vi "Read Dashboard Variables.vi"() -> ()   [LabVIEW 2018]
uses:
  <vilib>/Rock Robotics/Network Tables/NT Read Number.vi
  Framework/Robot Global Data.vi
panel:
  out "Elevator Cargo":dbl=2.0
  out "Elevator Hatch 3":dbl=2.0
  out "Elevator Hatch 2":dbl=2.0
  out "Elevator Hatch 1":dbl=2.0
  out "Elevator Ball 3":dbl=2.0
  out "Elevator Ball 2":dbl=2.0
  out "Elevator Ball 1":dbl=2.0
  out "Hatch Mover Scale":dbl=1.0 min=0.0 max=1.0 step=0.1
  out "Elevator Scale":dbl=1.0 min=0.0 max=1.0 step=0.1
  out "Autonomous Wait":u32=10
  out "Hatch Mover Duration":dbl=3.0
  out "Hatch Mover Setpoint":dbl=1.0
  out "SlowModeSettings":i32=2
  out "MaxSpeedSlow":dbl=0.4
  out "SlowRate":dbl=1.0
  out "MaxTurnSlow":dbl=0.55
  out "MaxTurnRateSlow":dbl=20.0
  out "Cargo Stop Current":dbl=10.0
  out "Cargo Hold Duration":dbl=1.0
  out "Cheezy Drive Mode":u32=2
  out "Cargo Setpoint":dbl=1.0 min=0.0 max=1.0 step=0.1
  out "Elevator Duration":dbl=2.0
  out "Elevator Setpoint":dbl=1.0 min=0.0 max=1.0 step=0.1
  out "Pivot Right Setpoint":dbl=0.3 min=0.0 max=1.0 step=0.1
  out "Pivot Left Setpoint":dbl=0.3 min=0.0 max=1.0 step=0.1
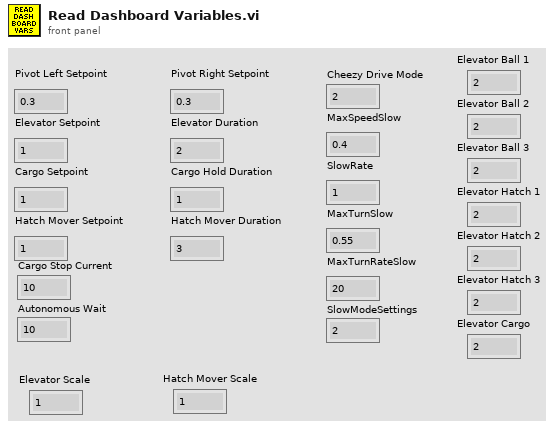
[diagram p1: front panel]
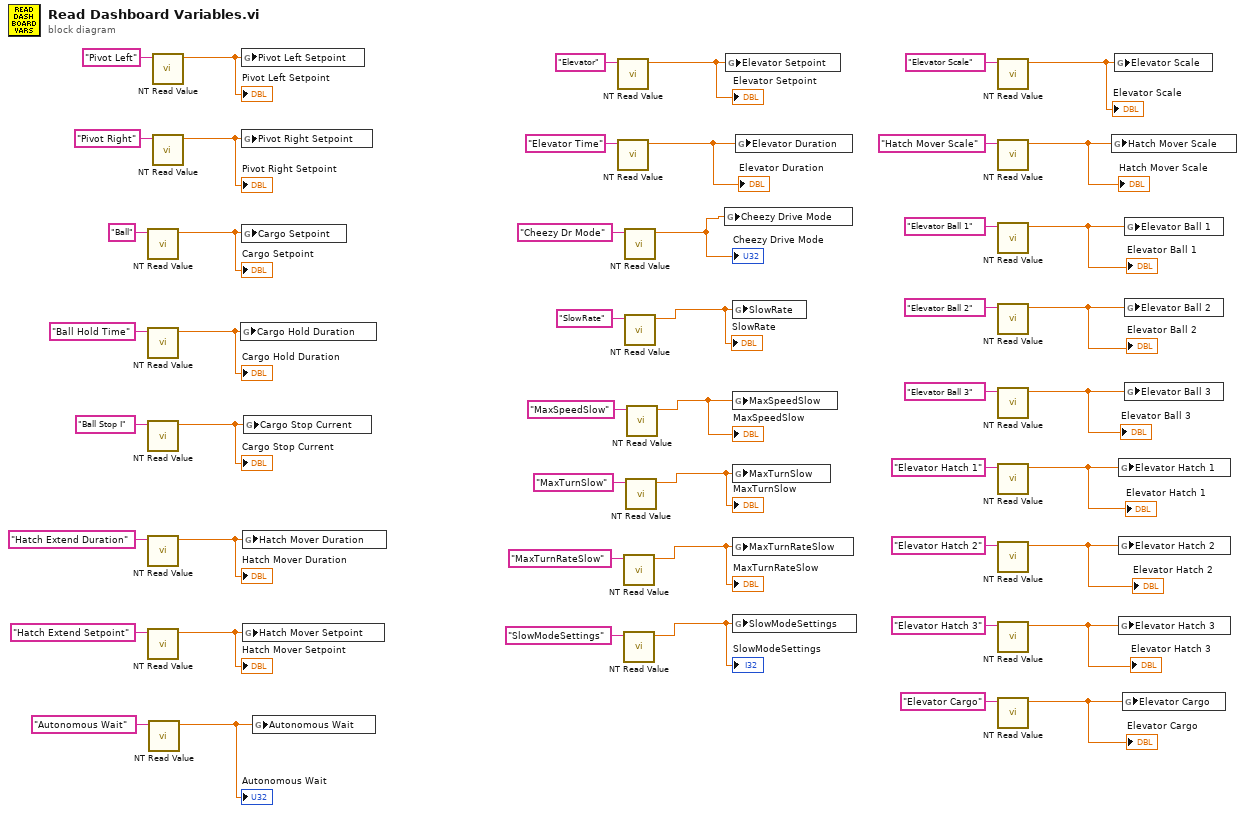
[diagram p0: block diagram]
diagram:
  n1 = call-poly <vilib>:"NT Read Value.vi"("Name"="Ball") -> ("Numeric"=w33:dbl)  [unwired: 9 in, 1 out]
  "Cargo Setpoint" <- w33
  n2 = call-poly <vilib>:"NT Read Value.vi"("Name"="Ball Hold Time") -> ("Numeric"=w32:dbl)  [unwired: 9 in, 1 out]
  "Cargo Hold Duration" <- w32
  n3 = call-poly <vilib>:"NT Read Value.vi"("Name"="Ball Stop I") -> ("Numeric"=w31:dbl)  [unwired: 9 in, 1 out]
  "Cargo Stop Current" <- w31
  n4 = call-poly <vilib>:"NT Read Value.vi"("Name"="Hatch Extend Duration") -> ("Numeric"=w30:dbl)  [unwired: 9 in, 1 out]
  "Hatch Mover Duration" <- w30
  n5 = call-poly <vilib>:"NT Read Value.vi"("Name"="Hatch Extend Setpoint") -> ("Numeric"=w29:dbl)  [unwired: 9 in, 1 out]
  "Hatch Mover Setpoint" <- w29
  n6 = call-poly <vilib>:"NT Read Value.vi"("Name"="Autonomous Wait") -> ("Numeric"=w20:dbl)  [unwired: 9 in, 1 out]
  "Autonomous Wait" <- w20
  n7 = call-poly <vilib>:"NT Read Value.vi"("Name"="Pivot Left") -> ("Numeric"=w35:dbl)  [unwired: 9 in, 1 out]
  "Pivot Left Setpoint" <- w35
  n8 = call-poly <vilib>:"NT Read Value.vi"("Name"="Pivot Right") -> ("Numeric"=w34:dbl)  [unwired: 9 in, 1 out]
  "Pivot Right Setpoint" <- w34
  n9 = global write "Robot Global Data.vi" "Cargo Hold Duration"(w32) -> ()
  n10 = global write "Robot Global Data.vi" "Pivot Left Setpoint"(w35) -> ()
  n11 = global write "Robot Global Data.vi" "Pivot Right Setpoint"(w34) -> ()
  n12 = global write "Robot Global Data.vi" "Cargo Setpoint"(w33) -> ()
  n13 = global write "Robot Global Data.vi" "Hatch Mover Duration"(w30) -> ()
  n14 = global write "Robot Global Data.vi" "Hatch Mover Setpoint"(w29) -> ()
  n15 = global write "Robot Global Data.vi" "Cargo Stop Current"(w31) -> ()
  n16 = global write "Robot Global Data.vi" "Autonomous Wait"(w20) -> ()
  n17 = call-poly <vilib>:"NT Read Value.vi"("Name"="Elevator") -> ("Numeric"=w22:dbl)  [unwired: 9 in, 1 out]
  "Elevator Setpoint" <- w22
  n18 = call-poly <vilib>:"NT Read Value.vi"("Name"="Elevator Time") -> ("Numeric"=w8:dbl)  [unwired: 9 in, 1 out]
  "Elevator Duration" <- w8
  n19 = call-poly <vilib>:"NT Read Value.vi"("Name"="MaxTurnRateSlow") -> ("Numeric"=w24:dbl)  [unwired: 9 in, 1 out]
  "MaxTurnRateSlow" <- w24
  n20 = call-poly <vilib>:"NT Read Value.vi"("Name"="SlowModeSettings") -> ("Numeric"=w23:dbl)  [unwired: 9 in, 1 out]
  "SlowModeSettings" <- w23
  n21 = call-poly <vilib>:"NT Read Value.vi"("Name"="Cheezy Dr Mode") -> ("Numeric"=w28:dbl)  [unwired: 9 in, 1 out]
  "Cheezy Drive Mode" <- w28
  n22 = call-poly <vilib>:"NT Read Value.vi"("Name"="SlowRate") -> ("Numeric"=w27:dbl)  [unwired: 9 in, 1 out]
  "SlowRate" <- w27
  n23 = call-poly <vilib>:"NT Read Value.vi"("Name"="MaxTurnSlow") -> ("Numeric"=w25:dbl)  [unwired: 9 in, 1 out]
  "MaxTurnSlow" <- w25
  n24 = call-poly <vilib>:"NT Read Value.vi"("Name"="MaxSpeedSlow") -> ("Numeric"=w26:dbl)  [unwired: 9 in, 1 out]
  "MaxSpeedSlow" <- w26
  n25 = global write "Robot Global Data.vi" "Cheezy Drive Mode"(w28) -> ()
  n26 = global write "Robot Global Data.vi" "Elevator Setpoint"(w22) -> ()
  n27 = global write "Robot Global Data.vi" "SlowRate"(w27) -> ()
  n28 = global write "Robot Global Data.vi" "MaxSpeedSlow"(w26) -> ()
  n29 = global write "Robot Global Data.vi" "MaxTurnSlow"(w25) -> ()
  n30 = global write "Robot Global Data.vi" "MaxTurnRateSlow"(w24) -> ()
  n31 = global write "Robot Global Data.vi" "SlowModeSettings"(w23) -> ()
  n32 = global write "Robot Global Data.vi" "Elevator Duration"(w8) -> ()
  n33 = call-poly <vilib>:"NT Read Value.vi"("Name"="Elevator Scale") -> ("Numeric"=w17:dbl)  [unwired: 9 in, 1 out]
  "Elevator Scale" <- w17
  n34 = call-poly <vilib>:"NT Read Value.vi"("Name"="Hatch Mover Scale") -> ("Numeric"=w16:dbl)  [unwired: 9 in, 1 out]
  "Hatch Mover Scale" <- w16
  n35 = call-poly <vilib>:"NT Read Value.vi"("Name"="Elevator Ball 1") -> ("Numeric"=w7:dbl)  [unwired: 9 in, 1 out]
  "Elevator Ball 1" <- w7
  n36 = call-poly <vilib>:"NT Read Value.vi"("Name"="Elevator Ball 2") -> ("Numeric"=w6:dbl)  [unwired: 9 in, 1 out]
  "Elevator Ball 2" <- w6
  n37 = call-poly <vilib>:"NT Read Value.vi"("Name"="Elevator Ball 3") -> ("Numeric"=w5:dbl)  [unwired: 9 in, 1 out]
  "Elevator Ball 3" <- w5
  n38 = call-poly <vilib>:"NT Read Value.vi"("Name"="Elevator Hatch 1") -> ("Numeric"=w4:dbl)  [unwired: 9 in, 1 out]
  "Elevator Hatch 1" <- w4
  n39 = call-poly <vilib>:"NT Read Value.vi"("Name"="Elevator Hatch 2") -> ("Numeric"=w3:dbl)  [unwired: 9 in, 1 out]
  "Elevator Hatch 2" <- w3
  n40 = call-poly <vilib>:"NT Read Value.vi"("Name"="Elevator Hatch 3") -> ("Numeric"=w2:dbl)  [unwired: 9 in, 1 out]
  "Elevator Hatch 3" <- w2
  n41 = call-poly <vilib>:"NT Read Value.vi"("Name"="Elevator Cargo") -> ("Numeric"=w1:dbl)  [unwired: 9 in, 1 out]
  "Elevator Cargo" <- w1
  n42 = global write "Robot Global Data.vi" "Hatch Mover Scale"(w16) -> ()
  n43 = global write "Robot Global Data.vi" "Elevator Scale"(w17) -> ()
  n44 = global write "Robot Global Data.vi" "Elevator Hatch 1"(w4) -> ()
  n45 = global write "Robot Global Data.vi" "Elevator Hatch 2"(w3) -> ()
  n46 = global write "Robot Global Data.vi" "Elevator Hatch 3"(w2) -> ()
  n47 = global write "Robot Global Data.vi" "Elevator Cargo"(w1) -> ()
  n48 = global write "Robot Global Data.vi" "Elevator Ball 1"(w7) -> ()
  n49 = global write "Robot Global Data.vi" "Elevator Ball 2"(w6) -> ()
  n50 = global write "Robot Global Data.vi" "Elevator Ball 3"(w5) -> ()
